vi "EstimateStates.vi"(8 "error in (no error)":errorcluster, 10 "Vessel In":refnum<class "Vessel.lvclass">, 11 "Attitude Observer in":refnum<class "Attitude Observer.lvclass">) -> (0 "error out":errorcluster, 2 "Vessel Out":refnum<class "Vessel.lvclass">, 3 "Attitude Observer out":refnum<class "Attitude Observer.lvclass">)   [LabVIEW 2014, in "Observer Library.lvlib" / "Attitude Observer.lvclass"]
uses:
  Attitude Observer.lvclass
  ROV/Vessel.lvclass
  <vilib>/Analysis/Matrix/Datatypes/RealMatrix.ctl
  Attitude Observer.lvclass/Attitude Observer.ctl
  Supervisor/Supervisor.lvclass
  <vilib>/Analysis/Matrix/NI_Matrix.lvlib
panel:
  in  "Fast":bool
  in  "k measured":dbl[](array[numeric])=[1.0, 1.0]
  in  "Ki":T1=[[0.005, 0.0, 0.0], [0.0, 0.005, 0.0], [0.0, 0.0, 0.005]]
  in  "Kp":T1=[[0.3, 0.0, 0.0], [0.0, 0.3, 0.0], [0.0, 0.0, 9.0]]
  in  "deviation":dbl
  in  "MTi_Theta_off":dbl[](array[numeric])=[0.0, 0.0, 0.0]
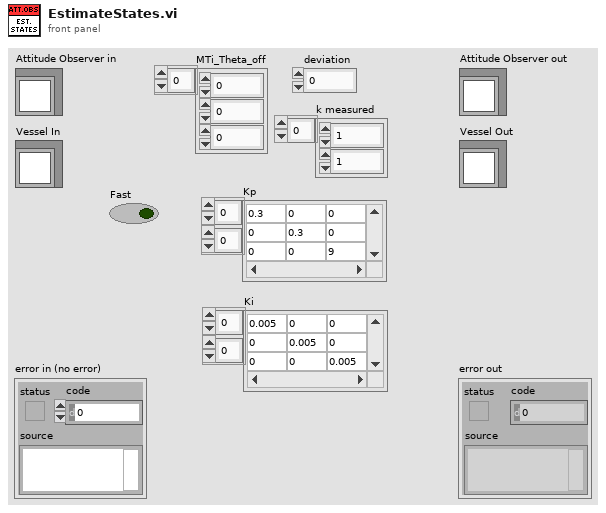
[diagram p1: front panel]
types:
  T1 = typedef "NI_Matrix.lvlib/RealMatrix.ctl" = dbl[][]
  T2 = cluster{"Measured":cluster{"Eta":dbl[], "Nu":dbl[], "Eta Dot":dbl[], "Nu Dot":dbl[]}, "Estimated":cluster{"Eta":dbl[], "Nu":dbl[], "Eta Dot":dbl[], "Nu Dot":dbl[]}, "Desired":cluster{"Eta":dbl[], "Nu":dbl[], "Eta Dot":dbl[], "Nu Dot":dbl[]}, "Previous Desired":cluster{"Eta":dbl[], "Nu":dbl[], "Eta Dot":dbl[], "Nu Dot":dbl[]}, "tau":dbl[], "Altitude":cluster{"Measured":dbl, "Estimated":dbl, "Desired":dbl, "Previous Desired":dbl, "Approximated":dbl, "grad F":dbl[]}, "rpm":dbl[], "Attitude":cluster{"Theta Measured":dbl[], "Theta Estimated":dbl[], "Omega Measured":dbl[], "Omega Estimated":dbl[], "Gyro Bias":dbl[]}}
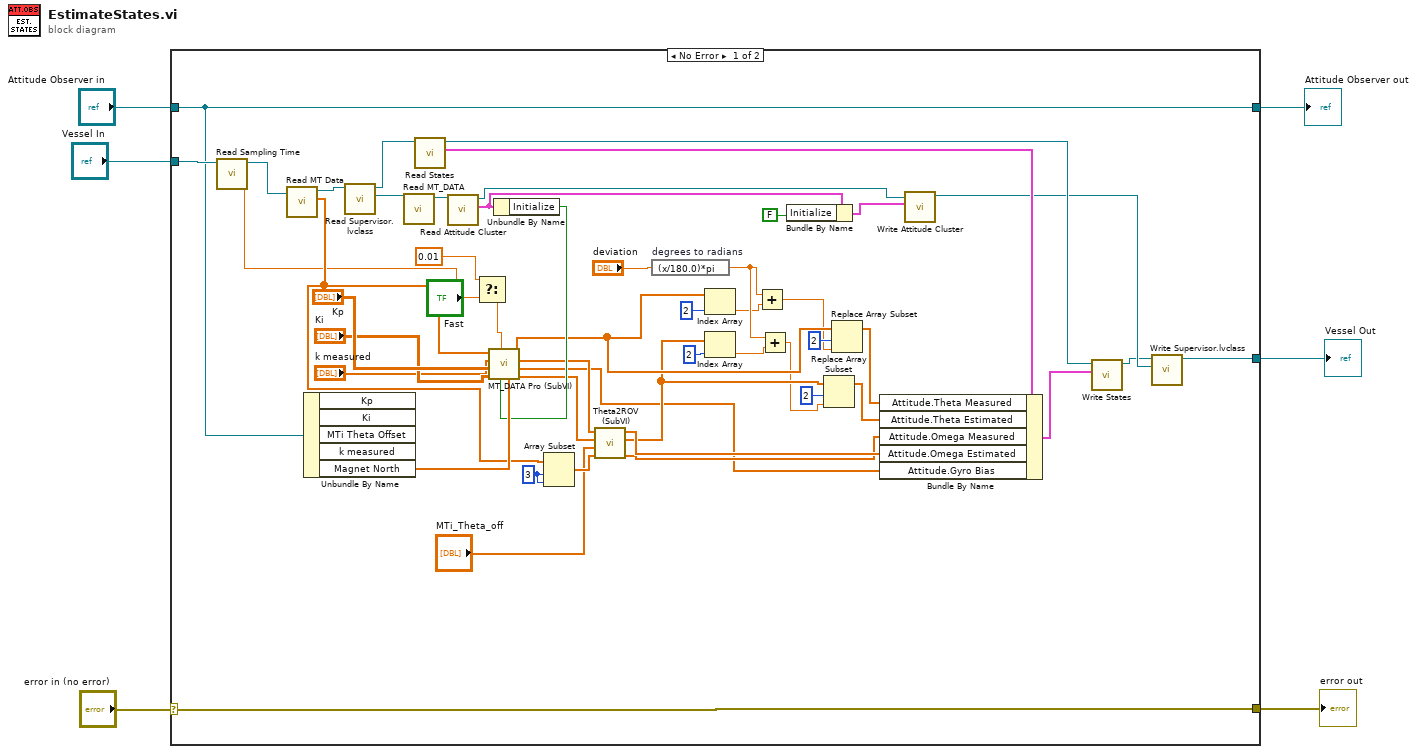
[diagram p0: block diagram]
diagram:
  n1 = case shown="No Error" "error in (no error)" {
    selector: "error in (no error)" -> [w34 w57]
    tunnel: "Vessel In" -> [w56 w58]
    tunnel: [w35 w58] -> w5
    tunnel: "Attitude Observer in" -> [w33 w59]
    tunnel: [w34 w57] -> w2
    tunnel: [w33 w59] -> w1
    frame No Error {
      w49 = 3 ("index")
      n2 = call-dynamic "Read Sampling Time.vi"("Vessel in"=w56) -> ("Sampling Time"=w10:dbl, "Vessel out"=w17:refnum<class "Vessel.lvclass">)  [unwired: 8 in, 1 out]
      n3 = call-dynamic "Read MT Data.vi"("Vessel in"=w17) -> ("MT Data"=w15:sgl[], "Vessel out"=w16:refnum<class "Vessel.lvclass">)  [unwired: 8 in, 1 out]
      n4 = Unbundle By Name(w33) -> ("Magnet North"=w55:dbl[])  [unwired: 4 out]
      n5 = call "Read Supervisor.lvclass.vi"("Vessel in"=w16) -> ("Supervisor.lvclass"=w54:refnum<class "Supervisor.lvclass">, "Vessel out"=w47:refnum<class "Vessel.lvclass">)  [unwired: 8 in, 1 out]
      n6 = call-dynamic "Read MT_DATA.vi"("Supervisor in"=w54) -> ("Supervisor out"=w53:refnum<class "Supervisor.lvclass">)  [unwired: 8 in, 2 out]
      n7 = call-dynamic "Read States.vi"("Vessel in"=w47) -> ("States"=w46:T2, "Vessel out"=w42:refnum<class "Vessel.lvclass">)  [unwired: 8 in, 1 out]
      n8 = call-dynamic "Read Attitude Cluster.vi"("Supervisor in"=w53) -> ("Attitude Cluster"=w41:cluster{"Initialize":bool}, "Supervisor out"=w38:refnum<class "Supervisor.lvclass">)  [unwired: 8 in, 1 out]
      n9 = Select(t=0.01 ("h"), s="Fast", f=w10) -> (s? t:f=w8:dbl)
      n10 = Unbundle By Name(w41) -> ("Initialize"=w52:bool)
      n11 = call "MT_DATA Pro (SubVI).vi"("mag_n"=w55, "Initialize"=w52, "h"=w8, "K_i"="Ki", "K_p"="Kp", "k_mes"="k measured", "MT_SINGLE"=w15) -> ("THETA_hat"=w51:dbl[], "bg"=w11:dbl[], "omega_hat"=w50:dbl[], "THETA_mes"=w25:dbl[])
      n12 = Array Subset(array=w15, index=w49, length=w49) -> (w48:sgl[])
      n13 = call "Theta2ROV (SubVI).vi"("omega_mti"=w48, "MTi_Theta_off"="MTi_Theta_off", "THETA_hat"=w51, "omega_hat"=w50) -> ("omega_rov_non_filtered"=w44:dbl[], "THETA_rov"=w20:dbl[], "omega_rov"=w45:dbl[])  [unwired: 5 in]
      n14 = expression code="(x/180.0)*pi" "degrees to radians"("deviation") -> (w28:dbl)
      n15 = Index Array(array=w25, index=2) -> (element=w27:dbl)
      n16 = Index Array(array=w20, index=2) -> (element=w26:dbl)
      n17 = Add(x=w28, y=w27) -> (x+y=w22:dbl)
      n18 = Add(x=w28, y=w26) -> (x+y=w18:dbl)
      n19 = Bundle By Name(cluster=w41, "Initialize"=FALSE) -> (w39:cluster{"Initialize":bool})
      n20 = Replace Array Subset(array=w20, new element=w18, index=2) -> (w19:dbl[])
      n21 = Replace Array Subset(array=w25, new element=w22, index=2) -> (w24:dbl[])
      n22 = Bundle By Name(cluster=w46, "Attitude.Theta Measured"=w24, "Attitude.Theta Estimated"=w19, "Attitude.Omega Measured"=w44, "Attitude.Omega Estimated"=w45, "Attitude.Gyro Bias"=w11) -> (w43:T2)
      n23 = call-dynamic "Write Attitude Cluster.vi"("Attitude Cluster"=w39, "Supervisor in"=w38) -> ("Supervisor out"=w37:refnum<class "Supervisor.lvclass">)  [unwired: 8 in, 1 out]
      n24 = call-dynamic "Write States.vi"("States"=w43, "Vessel in"=w42) -> ("Vessel out"=w36:refnum<class "Vessel.lvclass">)  [unwired: 8 in, 1 out]
      n25 = call "Write Supervisor.lvclass.vi"("Supervisor.lvclass"=w37, "Vessel in"=w36) -> ("Vessel out"=w35:refnum<class "Vessel.lvclass">)  [unwired: 8 in, 1 out]
    }
    frame Error {
    }
  }
  "error out" <- w2
  "Attitude Observer out" <- w1
  "Vessel Out" <- w5
